vi "SubVI server deposit.vi"(9 "before match":string, 10 "after match":string, 11 "appended path":path) -> (3 "String":string)   [LabVIEW 2020]
uses:
  <vilib>/Utility/file.llb/Read Delimited Spreadsheet (string).vi
  <vilib>/Utility/file.llb/Write Delimited Spreadsheet (string).vi
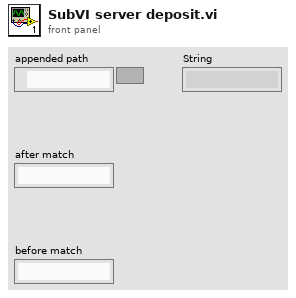
[diagram p1: front panel]
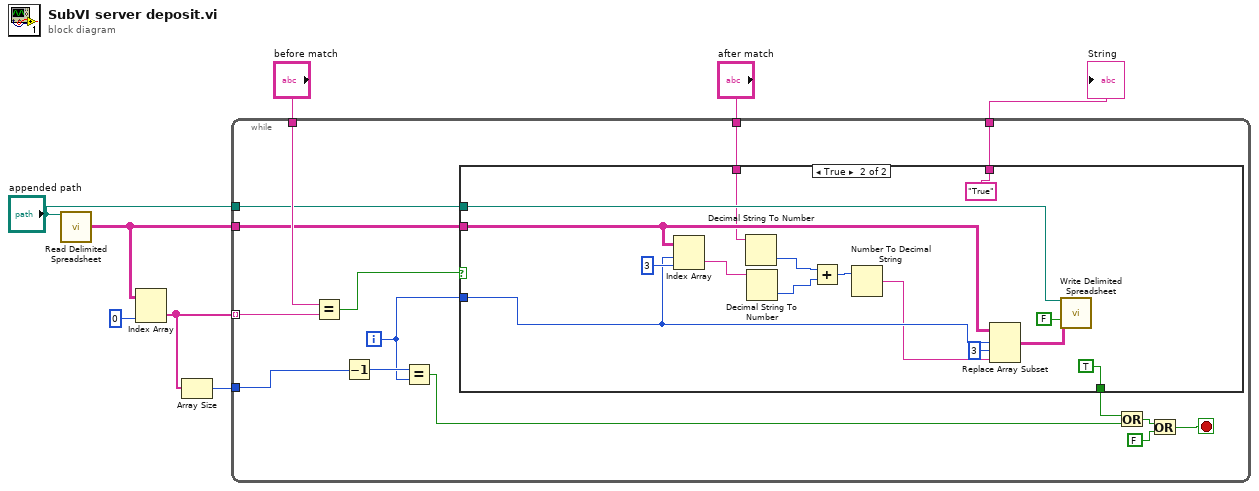
[diagram p0: block diagram]
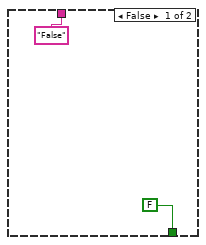
[diagram p2: hidden frame]
diagram:
  n1 = call-poly <vilib>:"Read Delimited Spreadsheet.vi"("file path (dialog if empty)"="appended path") -> ("all rows"=w2:string[][])  [unwired: 9 in, 5 out]
  n2 = Index Array "Index Array"(array=w2, index (col)=0 ("disabled index (col)")) -> (element=w3:string[])  [unwired: 1 in]
  n3 = Array Size(array=w3) -> (size(s)=w4:i32)
  n4 = while {
    tunnel: w2 -> [w18]
    tunnel: w3 -> [w15] mode=indexing
    tunnel: "before match" -> [w20]
    tunnel: w4 -> [w17]
    tunnel: "appended path" -> [w14]
    tunnel: [w13] -> w7
    tunnel: "after match" -> [w12]
    i -> [w16]
    stop <- w21 stop-if-true
    n5 = Equal?(x=w20, y=w15) -> (x = y?=w19:bool)
    n6 = Decrement(x=w17) -> (x-1=w22:i32)
    n7 = Equal?(x=w22, y=w16) -> (x = y?=w10:bool)
    n8 = case shown="True" w19 {
      tunnel: w18 -> [_ w37]
      tunnel: w16 -> [_ w33]
      tunnel: w14 -> [_ w40]
      tunnel: ["False" "True"] -> w13
      tunnel: w12 -> [_ w34]
      tunnel: [FALSE TRUE] -> w9
      frame False {
      }
      frame True {
        n9 = Index Array "Index Array"(array=w37, index (row)=w33, index (col)=3 ("disabled index (col)")) -> (element=w35:string)
        n10 = Decimal String To Number(string=w34) -> (number=w32:i32)  [unwired: 2 in, 1 out]
        n11 = Decimal String To Number(string=w35) -> (number=w31:i32)  [unwired: 2 in, 1 out]
        n12 = Add(x=w32, y=w31) -> (x+y=w30:i32)
        n13 = Number To Decimal String(number=w30) -> (decimal integer string=w27:string)  [unwired: 1 in]
        n14 = Replace Array Subset(array=w37, new element=w27, index (row)=w33, index (col)=3 ("disabled index (col)")) -> (w39:string[][])
        n15 = call-poly <vilib>:"Write Delimited Spreadsheet.vi"("file path (dialog if empty)"=w40, "2D data"=w39, "append to file? (new file:F)"=FALSE) -> ()  [unwired: 11 in, 2 out]
      }
    }
    n16 = Or(x=w9, y=w10) -> (x .or. y?=w11:bool)
    n17 = Or(x=w11, y=FALSE) -> (x .or. y?=w21:bool)
  }
  "String" <- w7
